vi "HMI_SelectArrayElement.vi"() -> ()   [LabVIEW 2024]
uses:
  <vilib>/Utility/miscctls.llb/LVPoint32TypeDef.ctl
panel:
  in  "File Type extension":string=".txt"
  out "Numeric":i32
  out "Coords":T1
  in  "stop":bool
  out "Array":string[](array[string])
  out "path":path
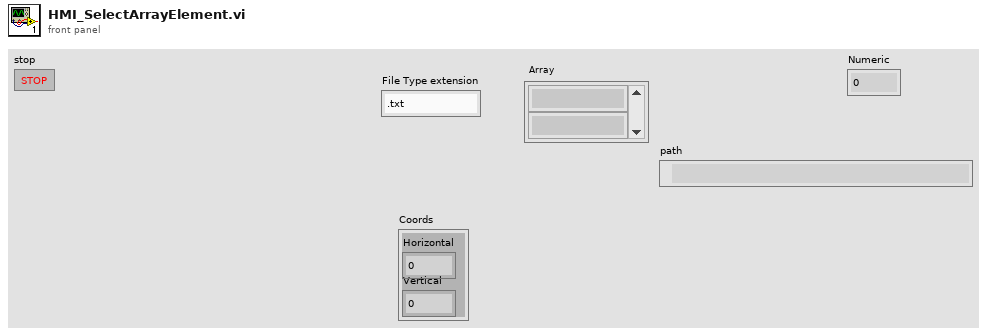
[diagram p1: front panel]
types:
  T1 = typedef "LVPoint32TypeDef.ctl" = cluster{"Horizontal":i32, "Vertical":i32}
  T2 = typedef "LVBoundsTypeDef.ctl" = cluster{"Width":u32, "Height":u32}
  T3 = typedef "LVRectTypeDef.ctl" = cluster{"Left":i16, "Top":i16, "Right":i16, "Bottom":i16}
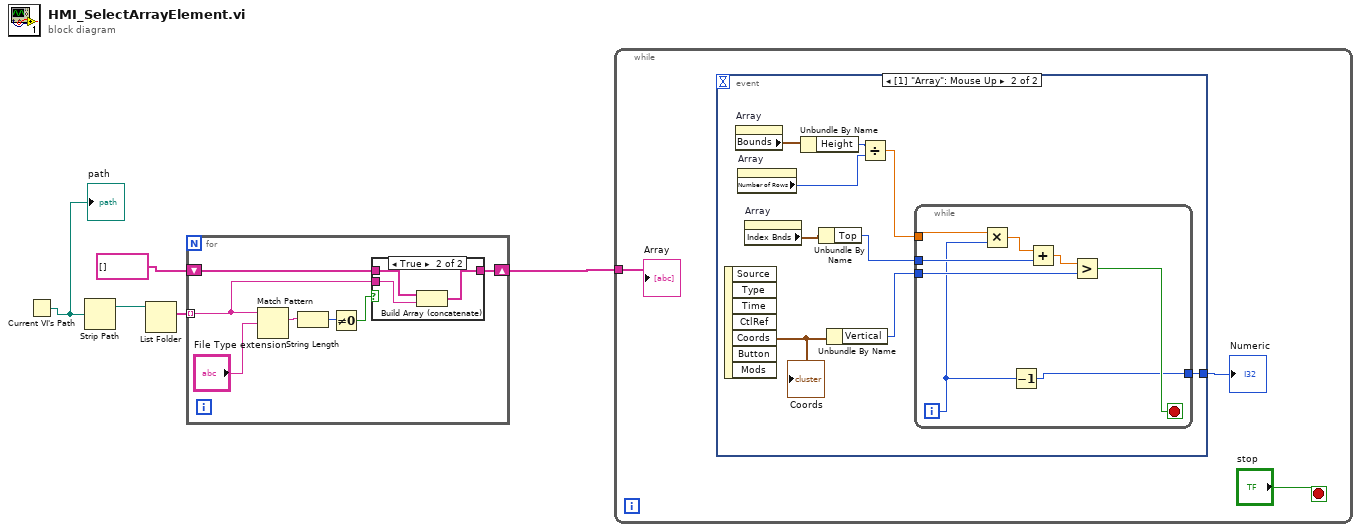
[diagram p0: block diagram]
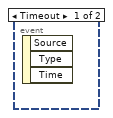
[diagram p2: hidden frame]
diagram:
  n1 = Current VI's Path() -> (path=w1:path)
  "path" <- w1
  n2 = Strip Path(path=w1) -> (stripped path=w5:path)  [unwired: 1 out]
  n3 = List Folder(path=w5) -> (filenames=w4:string[])  [unwired: 3 in, 3 out]
  n4 = for {
    tunnel: w4 -> [w6] mode=indexing
    shift-right: [w8] -> w2
    shift-left: string[] [] ("Array") -> [w7]
    n5 = Match Pattern(string=w6, regular expression="File Type extension") -> (match substring=w11:string)  [unwired: 1 in, 3 out]
    n6 = String Length(string=w11) -> (length=w10:i32)
    n7 = Not Equal To 0?(x=w10) -> (x != 0?=w9:bool)
    n8 = case shown="True" w9 {
      tunnel: [w13 w14] -> w8
      tunnel: w7 -> [w13 w16]
      tunnel: w6 -> [_ w15]
      frame False {
      }
      frame True {
        n9 = Build Array (concatenate)(w16, w15) -> (w14:string[])
      }
    }
  }
  n10 = while {
    tunnel: w2 -> [w19]
    stop <- "stop" stop-if-true
    n11 = event shown="[1] \"Array\": Mouse Up" {
      selector: _ -> [_ _]
      dyn-events: _ -> [_ _]
      timeout: _ -> [_ _]
      tunnel: [_ w20] -> w17
      event Timeout {
        n12 = event-data() -> ()  [unwired: 1 in, 3 out]
      }
      event "Array": Mouse Up {
        n13 = event-data() -> ("Coords"=w28:T1)  [unwired: 1 in, 6 out]
        "Coords" <- w28
        n14 = property on="Array" class="Arr (strict)"() -> ("Bounds"=w24:T2)  [unwired: 2 in, 2 out]
        n15 = property on="Array" class="Arr (strict)"() -> ("Number of Rows"=w25:u32)  [unwired: 2 in, 2 out]
        n16 = property on="Array" class="Arr (strict)"() -> ("Index Bnds"=w22:T3)  [unwired: 2 in, 2 out]
        n17 = Unbundle By Name(w24) -> ("Height"=w26:u32)
        n18 = Unbundle By Name(w22) -> ("Top"=w21:i16)
        n19 = Unbundle By Name(w28) -> ("Vertical"=w27:i32)
        n20 = Divide(x=w26, y=w25) -> (x/y=w23:dbl)
        n21 = while {
          tunnel: w21 -> [w34]
          tunnel: w23 -> [w36]
          tunnel: w27 -> [w32]
          tunnel: [w29] -> w20
          i -> [w30]
          stop <- w31 stop-if-true
          n22 = Multiply(x=w36, y=w30) -> (x*y=w35:dbl)
          n23 = Decrement(x=w30) -> (x-1=w29:i32)
          n24 = Add(x=w35, y=w34) -> (x+y=w33:dbl)
          n25 = Greater?(x=w33, y=w32) -> (0:w31:bool)
        }
      }
    }
    "Numeric" <- w17
    "Array" <- w19
  }
